vi "VisionExecute.v.vi"   [LabVIEW 2020]
uses:
  <vilib>/Rock Robotics/WPI/ThirdParty/PhotonPoseStrategy_ENUM.ctl
  <vilib>/Rock Robotics/WPI/ThirdParty/JAS_Junk/TrajLib/VI/Util_GetTime_U32.vi
  <vilib>/Rock Robotics/WPI/ThirdParty/PhotonVisionLib/SubVI/PhotonPipelineResult_CreateFromPacket.vi
  <vilib>/Rock Robotics/WPI/ThirdParty/PhotonVisionLib/SubVI/PhotonPipelineResult_SetTimeStampSecs.vi
  <vilib>/Rock Robotics/WPI/ThirdParty/PhotonVisionLib/SubVI/PhotonPipelineResult_GetLatency_Millis.vi
  <vilib>/Rock Robotics/WPI/ThirdParty/PhotonVisionLib/SubVI/PhotonPipelineResult_GetTimeStampSecs.vi
  <vilib>/Rock Robotics/WPI/ThirdParty/JAS_Junk/TrajLib/VI/Transform3d_Equals.vi
  <vilib>/Rock Robotics/WPI/ThirdParty/PhotonVisionLib/SubVI/PhotonPoseEstimator_SetStategy.vi
  <vilib>/Rock Robotics/WPI/ThirdParty/PhotonVisionLib/SubVI/PhotonPoseEstimator_SetHighestAmbiguity.vi
  <vilib>/Rock Robotics/WPI/ThirdParty/PhotonVisionLib/SubVI/PhotonPoseEstimator_New.vi
  <vilib>/Rock Robotics/WPI/ThirdParty/JAS_Junk/TrajLib/VI/AprilTagFieldLayout_NewSelect.vi
  <vilib>/Rock Robotics/WPI/ThirdParty/PhotonVisionLib/SubVI/PhotonPoseEstimator_SetLastPose.vi
  <vilib>/Rock Robotics/WPI/ThirdParty/PhotonVisionLib/SubVI/PhotonPoseEstimator_Update_PipeResult.vi
  <vilib>/Rock Robotics/WPI/ThirdParty/PhotonVisionLib/SubVI/PhotonPoseEstimator_SetReferencePose.vi
  <vilib>/Rock Robotics/WPI/ThirdParty/JAS_Junk/TrajLib/VI/Quaternion_New.vi
  <vilib>/Rock Robotics/WPI/ThirdParty/JAS_Junk/TrajLib/Conv_Deg_Radians.vi
  <vilib>/Rock Robotics/WPI/ThirdParty/JAS_Junk/TrajLib/VI/Pose3d_getTranslation3d.vi
  <vilib>/Rock Robotics/WPI/ThirdParty/JAS_Junk/TrajLib/VI/Pose3d_getRotation3d.vi
  <vilib>/Rock Robotics/WPI/ThirdParty/JAS_Junk/TrajLib/VI/Translation3d_ToTranslation2d.vi
  <vilib>/Rock Robotics/WPI/ThirdParty/JAS_Junk/TrajLib/VI/Rotation3d_ToRotation2d.vi
  <vilib>/Rock Robotics/WPI/ThirdParty/JAS_Junk/TrajLib/Pose2d_New_TRRO.vi
  <vilib>/Rock Robotics/WPI/ThirdParty/PhotonVisionLib/SubVI/Packet_decode_Flt64.vi
  <vilib>/Rock Robotics/WPI/ThirdParty/PhotonVisionLib/SubVI/Packet_decode_ByteI8.vi
  <vilib>/Rock Robotics/WPI/ThirdParty/PhotonVisionLib/SubVI/PhotonTrackedTarget_CreateFromPacket.vi
  <vilib>/Rock Robotics/WPI/ThirdParty/JAS_Junk/TrajLib/VI/Transform3d_GetTranslation3d.vi
  <vilib>/Rock Robotics/WPI/ThirdParty/JAS_Junk/TrajLib/VI/Transform3d_GetRotation3d.vi
  <vilib>/Rock Robotics/WPI/ThirdParty/JAS_Junk/TrajLib/VI/Rotation3d_Equals.vi
  <vilib>/Rock Robotics/WPI/ThirdParty/JAS_Junk/TrajLib/VI/Translation3d_Equals.vi
  <vilib>/Rock Robotics/WPI/ThirdParty/JAS_Junk/TrajLib/VI/AprilTagFieldLayout_New2022.vi
  <vilib>/Rock Robotics/WPI/ThirdParty/JAS_Junk/TrajLib/VI/AprilTagFieldLayout_New2023.vi
  <vilib>/Rock Robotics/WPI/ThirdParty/PhotonVisionLib/SubVI/PhotonPoseEstimator_GetEmptyPose.vi
  <vilib>/Rock Robotics/WPI/ThirdParty/PhotonVisionLib/SubVI/PhotonPoseEstimator_lowestAmbiguityStrategy.vi
  <vilib>/Rock Robotics/WPI/ThirdParty/PhotonVisionLib/SubVI/PhotonPoseEstimator_closestToCameraHeightStrategy.vi
  <vilib>/Rock Robotics/WPI/ThirdParty/PhotonVisionLib/SubVI/PhotonPoseEstimator_closestToReferencePoseStrategy.vi
  <vilib>/Rock Robotics/WPI/ThirdParty/PhotonVisionLib/SubVI/PhotonPoseEstimator_GetReferencePose.vi
  <vilib>/Rock Robotics/WPI/ThirdParty/PhotonVisionLib/SubVI/PhotonPoseEstimator_GetLastPose.vi
  <vilib>/Rock Robotics/WPI/ThirdParty/PhotonVisionLib/SubVI/PhotonPoseEstimator_averageBestTargetsStrategy.vi
  <vilib>/Rock Robotics/WPI/ThirdParty/JAS_Junk/TrajLib/Translation2d_Create.vi
  <vilib>/Rock Robotics/WPI/ThirdParty/JAS_Junk/TrajLib/Rotation2d_CreateAngle.vi
  <vilib>/Rock Robotics/WPI/ThirdParty/JAS_Junk/TrajLib/VI/Rotation3d_GetXYZ.vi
  <vilib>/Rock Robotics/WPI/ThirdParty/PhotonVisionLib/SubVI/TargetCorner_New.vi
  <vilib>/Rock Robotics/WPI/ThirdParty/PhotonVisionLib/SubVI/Packet_decode_Int32.vi
  <vilib>/Rock Robotics/WPI/ThirdParty/PhotonVisionLib/SubVI/Packet_decode_Transform3d.vi
  <vilib>/Rock Robotics/WPI/ThirdParty/JAS_Junk/TrajLib/VI/Rotation3d_GetQuaterion.vi
  <vilib>/Rock Robotics/WPI/ThirdParty/JAS_Junk/TrajLib/VI/Quaternion_Equals.vi
  <vilib>/Rock Robotics/WPI/ThirdParty/JAS_Junk/TrajLib/VI/AprilTagFieldLayout_New.vi
  <vilib>/Rock Robotics/WPI/ThirdParty/JAS_Junk/TrajLib/VI/Pose3d_New_Trans3dRot3d.vi
  <vilib>/Rock Robotics/WPI/ThirdParty/JAS_Junk/TrajLib/VI/Rotation3d_Create_Quaternion.vi
  <vilib>/Rock Robotics/WPI/ThirdParty/JAS_Junk/TrajLib/VI/AprilTag_New.vi
  <vilib>/Rock Robotics/WPI/ThirdParty/JAS_Junk/TrajLib/VI/Rotation3d_Create_AxisAngle.vi
  <vilib>/Rock Robotics/WPI/ThirdParty/JAS_Junk/TrajLib/VI/Pose3d_New.vi
  <vilib>/Rock Robotics/WPI/ThirdParty/PhotonVisionLib/SubVI/PhotonPipelineResult_HasTargets.vi
  <vilib>/Rock Robotics/WPI/ThirdParty/PhotonVisionLib/SubVI/PhotonEstimatedRobotPose_New.vi
  <vilib>/Rock Robotics/WPI/ThirdParty/PhotonVisionLib/SubVI/PhotonPipelineResult_GetTargets.vi
  <vilib>/Rock Robotics/WPI/ThirdParty/PhotonVisionLib/SubVI/PhotonTrackedTarget_GetPoseAmbiguity.vi
  <vilib>/Rock Robotics/WPI/ThirdParty/PhotonVisionLib/SubVI/PhotonTrackedTarget_GetFiducialId.vi
  <vilib>/Rock Robotics/WPI/ThirdParty/PhotonVisionLib/SubVI/PhotonPoseEstimator_GetFieldTags.vi
  <vilib>/Rock Robotics/WPI/ThirdParty/JAS_Junk/TrajLib/VI/AprilTagFieldLayout_GetTagPose.vi
  <vilib>/Rock Robotics/WPI/ThirdParty/JAS_Junk/TrajLib/VI/Pose3d_TransformBy.vi
  <vilib>/Rock Robotics/WPI/ThirdParty/PhotonVisionLib/SubVI/PhotonTrackedTarget_GetBestCameraToTarget.vi
  <vilib>/Rock Robotics/WPI/ThirdParty/JAS_Junk/TrajLib/VI/Transform3d_Inverse.vi
  <vilib>/Rock Robotics/WPI/ThirdParty/PhotonVisionLib/SubVI/PhotonPoseEstimator_GetHighestAmbiguity.vi
  <vilib>/Rock Robotics/WPI/ThirdParty/PhotonVisionLib/SubVI/PhotonPoseEstimator_GetRobotToCamera.vi
  <vilib>/Rock Robotics/WPI/ThirdParty/PhotonVisionLib/SubVI/PhotonPoseEstimator_closestToCameraHeightStrategy_calc.vi
  <vilib>/Rock Robotics/WPI/ThirdParty/PhotonVisionLib/SubVI/PhotonTrackedTarget_GetAltCameraToTarget.vi
  <vilib>/Rock Robotics/WPI/ThirdParty/PhotonVisionLib/SubVI/PhotonPoseEstimator_closestToReferencePoseStrategy_calc.vi
  <vilib>/Rock Robotics/WPI/ThirdParty/PhotonVisionLib/SubVI/PhotonPoseEstimator_averageBestTargetsStrategy_calc.vi
  <vilib>/Rock Robotics/WPI/ThirdParty/JAS_Junk/TrajLib/VI/Rotation3d_Plus.vi
  <vilib>/Rock Robotics/WPI/ThirdParty/JAS_Junk/TrajLib/VI/Translation3d_Plus.vi
  <vilib>/Rock Robotics/WPI/ThirdParty/JAS_Junk/TrajLib/VI/Translation3d_Times.vi
  <vilib>/Rock Robotics/WPI/ThirdParty/JAS_Junk/TrajLib/VI/Rotation3d_Times.vi
  <vilib>/Rock Robotics/WPI/ThirdParty/JAS_Junk/TrajLib/VI/Rotation3d_Create_Default.vi
  <vilib>/Rock Robotics/WPI/ThirdParty/JAS_Junk/TrajLib/VI/Translation3d_Create_Default.vi
  <vilib>/Rock Robotics/WPI/ThirdParty/JAS_Junk/TrajLib/VI/Quaternion_Get_All.vi
  <vilib>/Rock Robotics/WPI/ThirdParty/JAS_Junk/TrajLib/VI/Quaternion_Get_Vect.vi
  <vilib>/Rock Robotics/WPI/ThirdParty/JAS_Junk/TrajLib/VI/Quaternion_Get_W.vi
  <vilib>/Rock Robotics/WPI/ThirdParty/JAS_Junk/TrajLib/VI/AprilTag_GetAll.vi
  <vilib>/Rock Robotics/WPI/ThirdParty/JAS_Junk/TrajLib/VI/Quaternion_Normalize.vi
  <vilib>/Rock Robotics/WPI/ThirdParty/JAS_Junk/TrajLib/VI/Vector_Norm.vi
  <vilib>/Rock Robotics/WPI/ThirdParty/JAS_Junk/TrajLib/VecBuilder_ArrayBy1Fill.vi
  <vilib>/Rock Robotics/WPI/ThirdParty/JAS_Junk/TrajLib/VI/Pose3d_RelativeTo.vi
  <vilib>/Rock Robotics/WPI/ThirdParty/JAS_Junk/TrajLib/VI/Translation3d_RotateBy.vi
  <vilib>/Rock Robotics/WPI/ThirdParty/JAS_Junk/TrajLib/Transform2d_Create_TransRot.vi
  <vilib>/Rock Robotics/WPI/ThirdParty/JAS_Junk/TrajLib/VI/Rotation3d_UnaryMinus.vi
  <vilib>/Rock Robotics/WPI/ThirdParty/JAS_Junk/TrajLib/VI/Translation3d_UnaryMinus.vi
  <vilib>/Rock Robotics/WPI/ThirdParty/JAS_Junk/TrajLib/VI/Transform3d_GetXYZ.vi
  <vilib>/Rock Robotics/WPI/ThirdParty/JAS_Junk/TrajLib/VI/Pose3d_getXYZ.vi
  <vilib>/Rock Robotics/WPI/ThirdParty/PhotonVisionLib/SubVI/PhotonPoseEstimator_CalcDifference.vi
  <vilib>/Rock Robotics/WPI/ThirdParty/JAS_Junk/TrajLib/VI/Rotation3d_RotateBy.vi
  <vilib>/Rock Robotics/WPI/ThirdParty/JAS_Junk/TrajLib/VI/Translation3d_GetXYZ.vi
  <vilib>/Rock Robotics/WPI/ThirdParty/JAS_Junk/TrajLib/VI/Quaternion_New_Default.vi
  <vilib>/Rock Robotics/WPI/ThirdParty/JAS_Junk/TrajLib/MatBuilder_Create.vi
  <vilib>/Rock Robotics/WPI/ThirdParty/JAS_Junk/TrajLib/VI/Transform3d_Create_Pose3dPose3d.vi
  <vilib>/Rock Robotics/WPI/ThirdParty/JAS_Junk/TrajLib/VI/Quaternion_Times.vi
  <vilib>/Rock Robotics/WPI/ThirdParty/JAS_Junk/TrajLib/VI/Quaternion_Inverse.vi
  <vilib>/Rock Robotics/WPI/ThirdParty/JAS_Junk/TrajLib/VI/Translation3d_GetDistance.vi
  <vilib>/Rock Robotics/WPI/ThirdParty/JAS_Junk/TrajLib/VI/Translation3d_Minus.vi
  <vilib>/Rock Robotics/WPI/ThirdParty/JAS_Junk/TrajLib/VI/Rotation3d_Minus.vi
  <vilib>/Rock Robotics/SystemInterfaces/Utilities/FPGA_UtilitiesRead LocalTime.vi
  <vilib>/Rock Robotics/WPI/ThirdParty/JAS_Junk/TrajLib/VI/Util_GetTime_U64.vi
  <vilib>/Rock Robotics/Network Tables/NT Read Value.vi
  <vilib>/Rock Robotics/Network Tables/NT Read Raw.vi
  VisionGlobal.vi
  <vilib>/Rock Robotics/WPI/ThirdParty/JAS_Junk/TrajLib/Trajectory_Library.lvlib
  <vilib>/Rock Robotics/WPI/ThirdParty/PhotonVisionLib/PhotonVisionLib.lvlib
  <vilib>/Rock Robotics/WPI/ThirdParty/JAS_Junk/TrajLib/TypeDef/TRANSLATION2D.ctl
  <vilib>/Rock Robotics/WPI/ThirdParty/JAS_Junk/TrajLib/TypeDef/ROTATION2D.ctl
  <vilib>/Rock Robotics/WPI/ThirdParty/JAS_Junk/TrajLib/TypeDef/POSE2D.ctl
types:
  T1 = typedef "PhotonVisionLib.lvlib/PhotonPoseStrategy_ENUM.ctl" = enum16{"LOWEST_AMBIGUITY", "CLOSEST_TO_CAMERA_HEIGHT", "CLOSEST_TO_REFERENCE_POSE", "CLOSEST_TO_LAST_POSE", "AVERAGE_BEST_TARGETS"}
  T2 = typedef "Trajectory_Library.lvlib/TRANSLATION3D.ctl" = cluster{"X":dbl, "Y":dbl, "Z":dbl}
  T3 = typedef "Trajectory_Library.lvlib/ROTATION3D.ctl" = cluster{"Q_quaternion":T4}
  T4 = typedef "Trajectory_Library.lvlib/QUATERNION.ctl" = cluster{"R":dbl, "V":dbl[]}
  T5 = typedef "Trajectory_Library.lvlib/TRANSFORM3D.ctl" = cluster{"TRANSLATION3D":T2, "ROTATION3D":T3, "XF":bool}
  T6 = typedef "PhotonVisionLib.lvlib/PhotonPipelineResultType.ctl" = cluster{"TargetCount":i32, "Latency_MilliSec":dbl, "Targets":T7[], "TimeStampSec":dbl}
  T7 = typedef "PhotonVisionLib.lvlib/PhotonTrackedTargetType.ctl" = cluster{"Yaw":dbl, "Pitch":dbl, "Area":dbl, "Skew":dbl, "MinAreaRectCorners":T8[], "BestCameraToTarget":T5, "FiiducialId":i32, "AltCameraToTarget":T5, "PoseAmbiguity":dbl, "DetectedCorners":T8[]}
  T8 = typedef "PhotonVisionLib.lvlib/TargetCornerType.ctl" = cluster{"X":dbl, "Y":dbl}
  T9 = typedef "PhotonVisionLib.lvlib/PhotonPoseEstimator_Configuration.ctl" = cluster{"Strategy":T1, "Camera":string, "Initial Pose":T10, "AprilTagField":enum16{"2022 Rapid React", "2023 Charged Up"}, "HighestAmbiguity":dbl, "Use Custom Field":bool, "Custom AprilTag Field":T11, "RobotToCamera":T5}
  T10 = typedef "Trajectory_Library.lvlib/POSE3D.ctl" = cluster{"Translation3d":T2, "Rotation3d":T3}
  T11 = typedef "Trajectory_Library.lvlib/AprilTagFieldLayout.ctl" = cluster{"AprilTagMap":map{i32, T12}, "FieldLength":dbl, "FieldWidth":dbl, "OriginPosition ":T13, "OriginPose3d":T10}
  T12 = typedef "Trajectory_Library.lvlib/AprilTag.ctl" = cluster{"ID":i32, "POSE3D":T10}
  T13 = typedef "Trajectory_Library.lvlib/AprilTagFieldLayoutOrignPosition_ENUM.ctl" = enum16{"kBlueAllianceWallRightSide,", "kRedAllianceWallRightSide,"}
  T14 = typedef "PhotonVisionLib.lvlib/PhotonEstimatedRobotPoseType.ctl" = cluster{"EstimatedPose":T10, "TimeStamp_Seconds":dbl}
  T15 = typedef "Trajectory_Library.lvlib/POSE2D.ctl" = cluster{"TRANSLATION":T16, "ROTATION":T17}
  T16 = typedef "Trajectory_Library.lvlib/TRANSLATION2D.ctl" = cluster{"X":dbl, "Y":dbl}
  T17 = typedef "Trajectory_Library.lvlib/ROTATION2D.ctl" = cluster{"VALUE":dbl, "COS":dbl, "SIN":dbl}
  T18 = typedef "Trajectory_Library.lvlib/DIFF_DRIVE_POSE_EST2_CONFIG.ctl" = cluster{"TrackWidth_Meters":dbl, "Odom X std dev M":dbl, "Odom Y std dev M":dbl, "Odom Heading std dev Rad":dbl, "Vision X std dev M":dbl, "Vision Y std dev M":dbl, "Vision Heading std dev Rad":dbl}
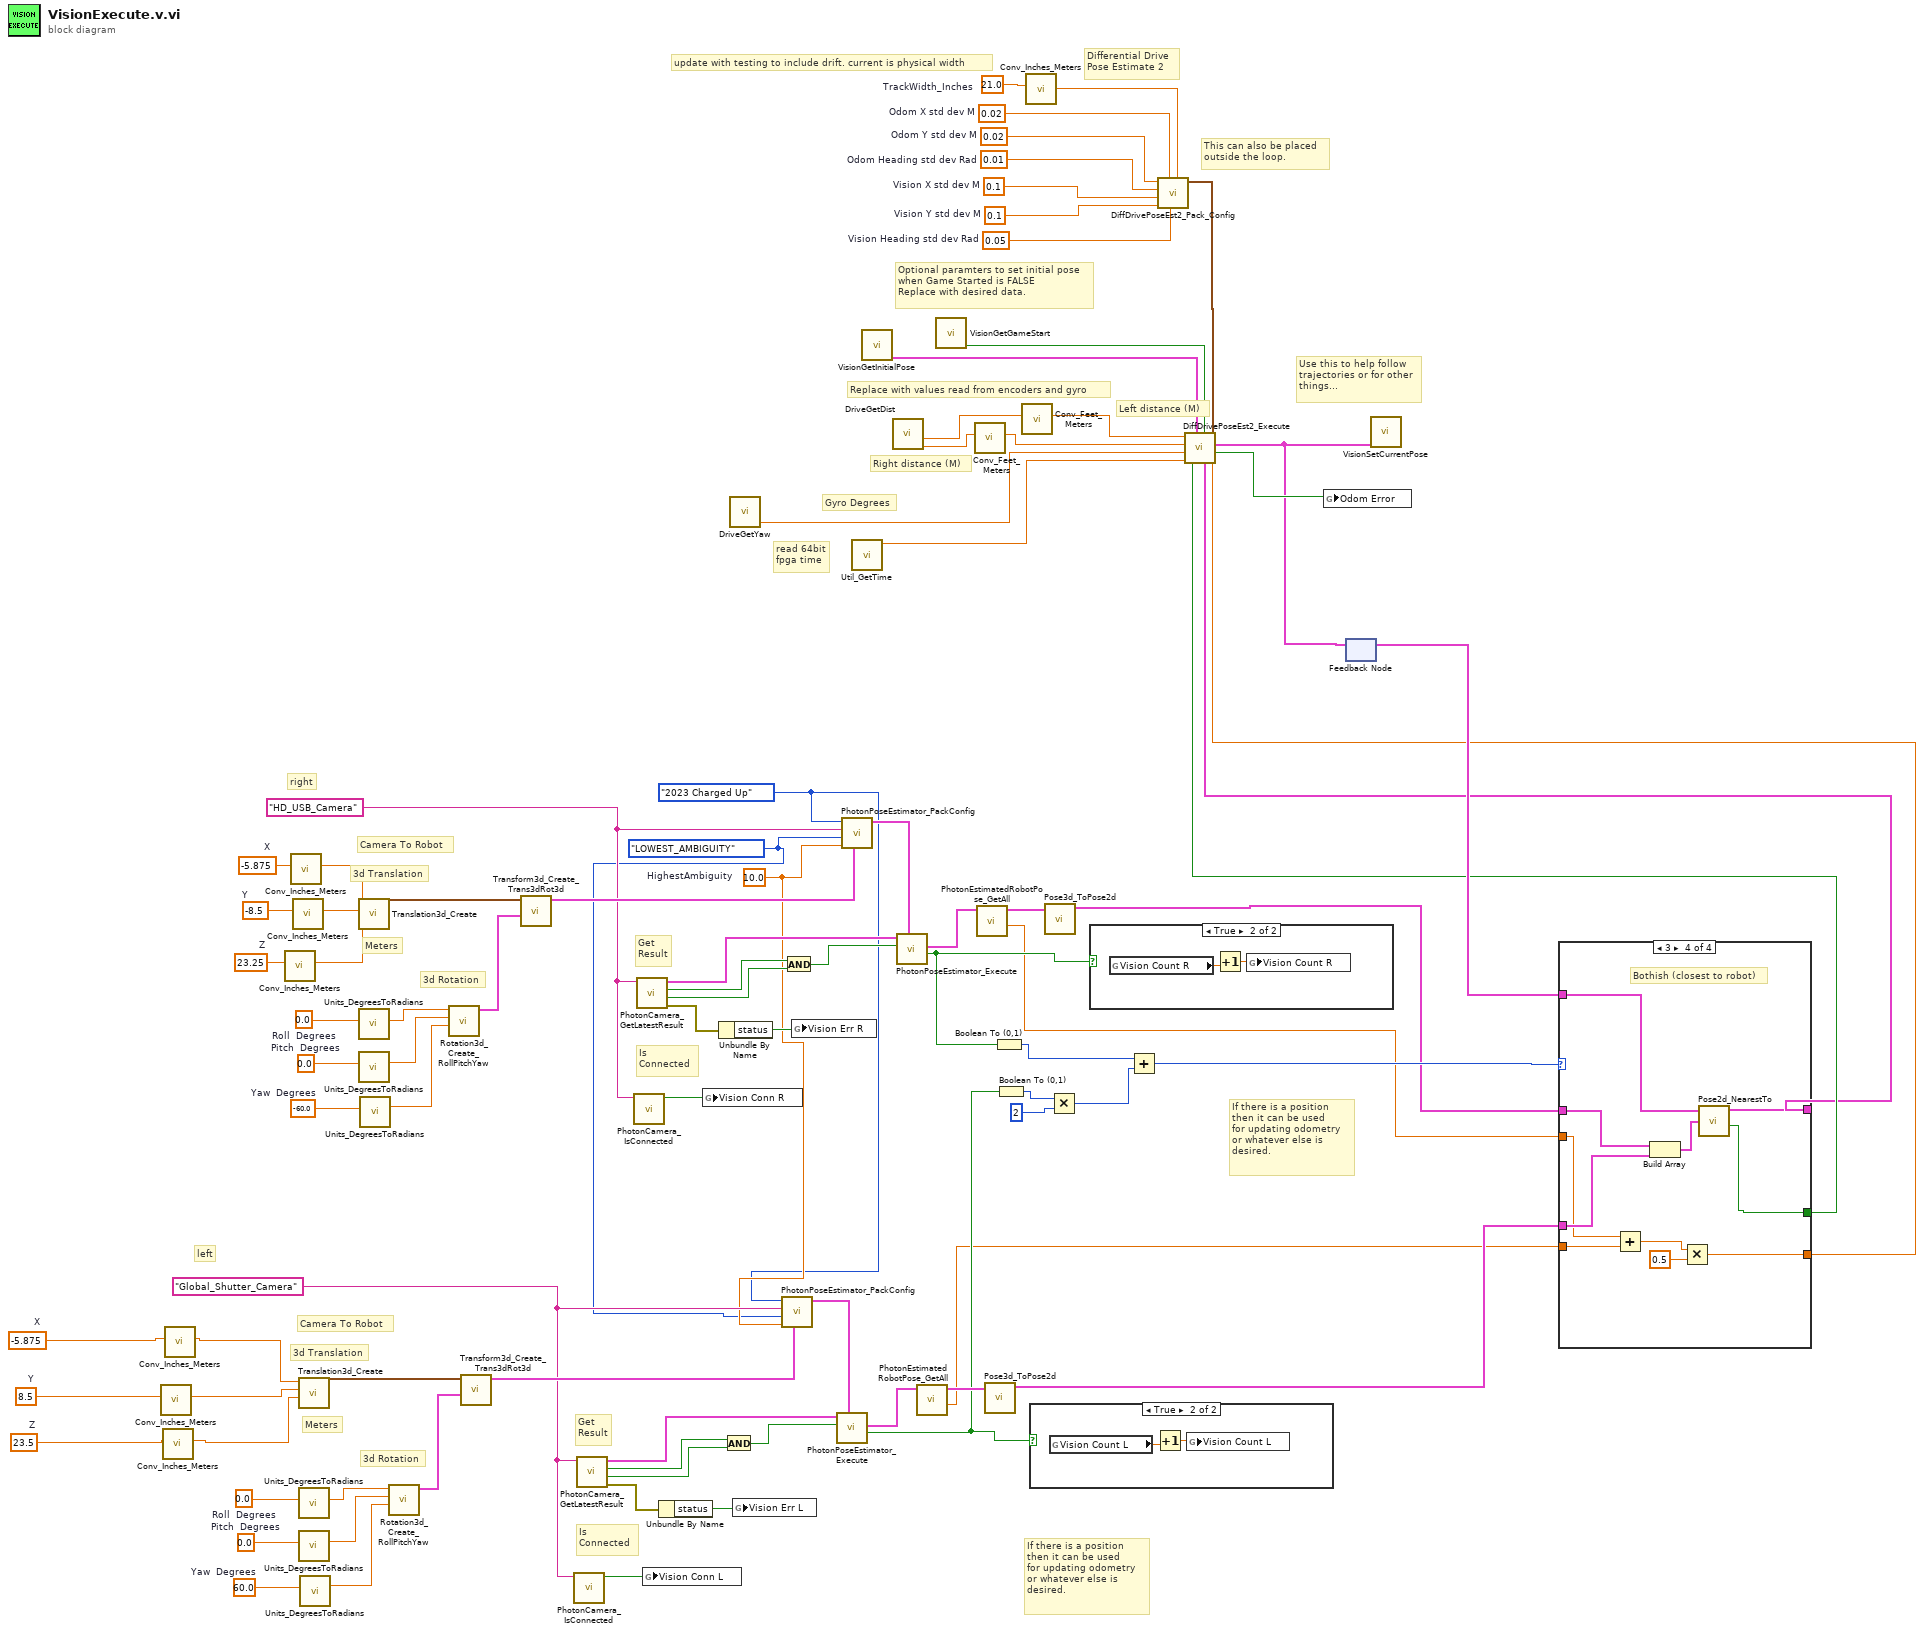
[diagram p0: block diagram]
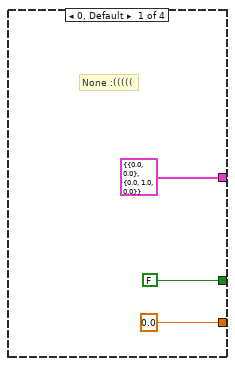
[diagram p2: hidden frame]
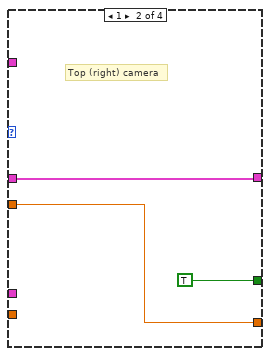
[diagram p3: hidden frame]
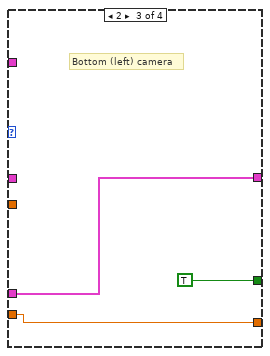
[diagram p4: hidden frame]
diagram:
  w44 = 0.0  # Roll  Degrees
  w43 = 0.0  # Pitch  Degrees
  w42 = 60.0  # Yaw  Degrees
  w27 = 23.5  # Z
  w31 = -5.875  # X
  w29 = 8.5  # Y
  w38 = "Global_Shutter_Camera" ("CameraName")
  w65 = 0.0  # Roll  Degrees
  w64 = 0.0  # Pitch  Degrees
  w63 = -60.0  # Yaw  Degrees
  w21 = 23.25  # Z
  w25 = -5.875  # X
  w23 = -8.5  # Y
  w19 = 10.0  # HighestAmbiguity
  w18 = PhotonPoseStrategy_ENUM."LOWEST_AMBIGUITY" ("Strategy")
  w17 = enum16{"2022 Rapid React", "2023 Charged Up"}."2023 Charged Up" ("AprilTagField")
  w59 = "HD_USB_Camera" ("CameraName")
  w81 = 21.0  # TrackWidth_Inches
  w83 = 0.02  # Odom Y std dev M
  w84 = 0.01  # Odom Heading std dev Rad
  w85 = 0.1  # Vision X std dev M
  w86 = 0.1  # Vision Y std dev M
  w87 = 0.02  # Odom X std dev M
  w88 = 0.05  # Vision Heading std dev Rad
  # "right"
  # "left"
  # "If there is a position\nthen it can be used\nfor updating odometry\nor whatever else is \ndesired."
  # "Meters"
  # "Camera To Robot"
  # "3d Rotation"
  # "3d Translation"
  # "Is\nConnected"
  # "Get\nResult"
  # "If there is a position\nthen it can be used\nfor updating odometry\nor whatever else is \ndesired."
  # "Meters"
  # "Camera To Robot"
  # "3d Rotation"
  # "3d Translation"
  # "Is\nConnected"
  # "Get\nResult"
  # "Gyro Degrees"
  # "Right distance (M)"
  # "Left distance (M)"
  # "update with testing to include drift. current is physical width"
  # "Replace with values read from encoders and gyro"
  # "Optional paramters to set initial pose\nwhen Game Started is FALSE\nReplace with desired data."
  # "read 64bit\nfpga time"
  # "This can also be placed \noutside the loop."
  # "Use this to help follow\ntrajectories or for other\nthings..."
  # "Differential Drive \nPose Estimate 2"
  n1 = call <vilib>:"Conv_Inches_Meters.vi"("INCH"=w29) -> ("Meters"=w28:dbl)  [unwired: 10 in]
  n2 = call <vilib>:"Conv_Inches_Meters.vi"("INCH"=w27) -> ("Meters"=w26:dbl)  [unwired: 10 in]
  n3 = call <vilib>:"Conv_Inches_Meters.vi"("INCH"=w31) -> ("Meters"=w30:dbl)  [unwired: 10 in]
  n4 = call <vilib>:"Conv_Inches_Meters.vi"("INCH"=w21) -> ("Meters"=w20:dbl)  [unwired: 10 in]
  n5 = call <vilib>:"Conv_Inches_Meters.vi"("INCH"=w25) -> ("Meters"=w24:dbl)  [unwired: 10 in]
  n6 = call <vilib>:"Conv_Inches_Meters.vi"("INCH"=w23) -> ("Meters"=w22:dbl)  [unwired: 10 in]
  n7 = call <vilib>:"Translation3d_Create.vi"("Z"=w26, "Y"=w28, "X"=w30) -> ("TRANSLATION3D"=w45:T2)  [unwired: 8 in]
  n8 = call <vilib>:"Units_DegreesToRadians.vi"("Degrees"=w44) -> ("Radians"=w41:dbl)  [unwired: 10 in]
  n9 = call <vilib>:"Units_DegreesToRadians.vi"("Degrees"=w43) -> ("Radians"=w40:dbl)  [unwired: 10 in]
  n10 = call <vilib>:"Units_DegreesToRadians.vi"("Degrees"=w42) -> ("Radians"=w39:dbl)  [unwired: 10 in]
  n11 = call <vilib>:"Translation3d_Create.vi"("Z"=w20, "Y"=w22, "X"=w24) -> ("TRANSLATION3D"=w66:T2)  [unwired: 8 in]
  n12 = call <vilib>:"Units_DegreesToRadians.vi"("Degrees"=w65) -> ("Radians"=w62:dbl)  [unwired: 10 in]
  n13 = call <vilib>:"Units_DegreesToRadians.vi"("Degrees"=w64) -> ("Radians"=w61:dbl)  [unwired: 10 in]
  n14 = call <vilib>:"Units_DegreesToRadians.vi"("Degrees"=w63) -> ("Radians"=w60:dbl)  [unwired: 10 in]
  n15 = call <vilib>:"Rotation3d_Create_RollPitchYaw.vi"("Yaw"=w39, "Pitch"=w40, "Roll"=w41) -> ("Rotation3d"=w46:T3)  [unwired: 8 in]
  n16 = call <vilib>:"Rotation3d_Create_RollPitchYaw.vi"("Yaw"=w60, "Pitch"=w61, "Roll"=w62) -> ("Rotation3d"=w67:T3)  [unwired: 8 in]
  n17 = call <vilib>:"Transform3d_Create_Trans3dRot3d.vi"("Rotation3d"=w46, "Translation3d"=w45) -> ("Transform3d"=w47:T5)  [unwired: 9 in]
  n18 = call <vilib>:"Transform3d_Create_Trans3dRot3d.vi"("Rotation3d"=w67, "Translation3d"=w66) -> ("Transform3d"=w68:T5)  [unwired: 9 in]
  n19 = call <vilib>:"PhotonCamera_IsConnected.vi"("CameraName"=w38) -> ("IsConnected"=w34:bool)  [unwired: 9 in, 1 out]
  n20 = call <vilib>:"PhotonCamera_GetLatestResult.vi"("CameraName"=w38) -> ("error out"=w33:errorcluster, "New Data"=w51:bool, "HasTargets"=w50:bool, "PipelineResult"=w48:T6)  [unwired: 7 in]
  n21 = call <vilib>:"PhotonCamera_IsConnected.vi"("CameraName"=w59) -> ("IsConnected"=w54:bool)  [unwired: 9 in, 1 out]
  n22 = call <vilib>:"PhotonCamera_GetLatestResult.vi"("CameraName"=w59) -> ("error out"=w53:errorcluster, "New Data"=w72:bool, "HasTargets"=w71:bool, "PipelineResult"=w69:T6)  [unwired: 7 in]
  n23 = global write "VisionGlobal.vi" "Vision Conn L"(w34) -> ()
  n24 = Unbundle By Name(w33) -> ("status"=w32:bool)
  n25 = global write "VisionGlobal.vi" "Vision Conn R"(w54) -> ()
  n26 = Unbundle By Name(w53) -> ("status"=w52:bool)
  n27 = And(x=w50, y=w51) -> (x .and. y?=w49:bool)
  n28 = call "DriveGetYaw.vi"() -> ("Yaw"=w75:dbl)  [unwired: 11 in]
  n29 = global write "VisionGlobal.vi" "Vision Err L"(w32) -> ()
  n30 = call <vilib>:"PhotonPoseEstimator_PackConfig.vi"("RobotToCamera"=w47, "HighestAmbiguity"=w19, "Strategy"=w18, "Camera"=w38, "AprilTagField"=w17) -> ("PoseEstimator_Configuration"=w37:T9)  [unwired: 6 in]
  n31 = And(x=w71, y=w72) -> (x .and. y?=w70:bool)
  n32 = global write "VisionGlobal.vi" "Vision Err R"(w52) -> ()
  n33 = call <vilib>:"PhotonPoseEstimator_Execute.vi"("Configuration"=w37, "PIpeline Has \nNew Results"=w49, "PipelineResult"=w48) -> ("Pos Found"=w14:bool, "PhotonEstimatedRobotPose"=w36:T14)  [unwired: 6 in, 1 out]
  n34 = call <vilib>:"PhotonPoseEstimator_PackConfig.vi"("RobotToCamera"=w68, "HighestAmbiguity"=w19, "Strategy"=w18, "Camera"=w59, "AprilTagField"=w17) -> ("PoseEstimator_Configuration"=w58:T9)  [unwired: 6 in]
  n35 = call <vilib>:"Util_GetTime.vi"() -> ("FPGA_Time_Seconds"=w82:dbl)  [unwired: 9 in, 2 out]
  n36 = call "VisionGetInitialPose.vi"() -> ("InitialPose"=w74:T15)  [unwired: 10 in]
  n37 = call "DriveGetDist.vi"() -> ("Right dist"=w79:dbl, "Left dist"=w78:dbl)  [unwired: 10 in]
  n38 = call <vilib>:"PhotonPoseEstimator_Execute.vi"("Configuration"=w58, "PIpeline Has \nNew Results"=w70, "PipelineResult"=w69) -> ("Pos Found"=w15:bool, "PhotonEstimatedRobotPose"=w57:T14)  [unwired: 6 in, 1 out]
  n39 = call <vilib>:"PhotonEstimatedRobotPose_GetAll.vi"("PhotonEstimatedRobotPose"=w36) -> ("TimeStamp_Seconds"=w4:dbl, "EstimatedPose"=w35:T10)  [unwired: 9 in]
  n40 = call "VisionGetGameStart.vi"() -> ("Game Start"=w73:bool)  [unwired: 11 in]
  n41 = call <vilib>:"Conv_Feet_Meters.vi"("Feet"=w79) -> ("Meters"=w76:dbl)  [unwired: 10 in]
  n42 = call <vilib>:"PhotonEstimatedRobotPose_GetAll.vi"("PhotonEstimatedRobotPose"=w57) -> ("TimeStamp_Seconds"=w5:dbl, "EstimatedPose"=w56:T10)  [unwired: 9 in]
  n43 = call <vilib>:"Pose3d_ToPose2d.vi"("in Pose3d"=w35) -> ("out Pose2d"=w7:T15)  [unwired: 10 in]
  n44 = Boolean To (0,1)(Boolean=w15) -> (0, 1=w10:i16)
  n45 = Boolean To (0,1)(Boolean=w14) -> (0, 1=w13:i16)
  n46 = call <vilib>:"Conv_Feet_Meters.vi"("Feet"=w78) -> ("Meters"=w77:dbl)  [unwired: 10 in]
  n47 = call <vilib>:"Conv_Inches_Meters.vi"("INCH"=w81) -> ("Meters"=w80:dbl)  [unwired: 10 in]
  n48 = case shown="True" w14 {
    frame False {
    }
    frame True {
      n49 = global read "VisionGlobal.vi" "Vision Count L"() -> (w90:dbl)
      n50 = Increment(x=w90) -> (x+1=w91:dbl)
      n51 = global write "VisionGlobal.vi" "Vision Count L"(w91) -> ()
    }
  }
  n52 = call <vilib>:"Pose3d_ToPose2d.vi"("in Pose3d"=w56) -> ("out Pose2d"=w8:T15)  [unwired: 10 in]
  n53 = Multiply(x=w13, y=i16 2) -> (x*y=w11:i16)
  n54 = case shown="True" w15 {
    frame False {
    }
    frame True {
      n55 = global read "VisionGlobal.vi" "Vision Count R"() -> (w92:dbl)
      n56 = Increment(x=w92) -> (x+1=w93:dbl)
      n57 = global write "VisionGlobal.vi" "Vision Count R"(w93) -> ()
    }
  }
  n58 = Add(x=w10, y=w11) -> (x+y=w9:i16)
  n59 = call <vilib>:"DiffDrivePoseEst2_Pack_Config.vi"("TrackWidth_Meters"=w80, "Vision Heading std dev Rad"=w88, "Odom X std dev M"=w87, "Vision Y std dev M"=w86, "Vision X std dev M"=w85, "Odom Heading std dev Rad"=w84, "Odom Y std dev M"=w83) -> ("DiffPoseEst2Config"=w89:T18)  [unwired: 4 in]
  n60 = feedback #1() -> (w6:T15)  [unwired: 1 in]
  n61 = case shown="3" w9 {
    tunnel: w8 -> [_ w98 _ w111]
    tunnel: w7 -> [_ _ w101 w110]
    tunnel: w6 -> [_ _ _ w112]
    tunnel: [FALSE ("Found") TRUE ("Found") TRUE ("Found") w108] -> w3
    tunnel: w5 -> [_ w99 _ w107]
    tunnel: w4 -> [_ _ w102 w106]
    tunnel: [T15 {"TRANSLATION"={"X"=0.0, "Y"=0.0}, "ROTATION"={"VALUE"=0.0, "COS"=1.0, "SIN"=0.0}} ("Nearest Pose") w98 w101 w109] -> w2
    tunnel: [0.0 w99 w102 w103] -> w1
    frame 0, Default {
      # "None :((((("
    }
    frame 1 {
      # "Top (right) camera"
    }
    frame 2 {
      # "Bottom (left) camera"
    }
    frame 3 {
      # "Bothish (closest to robot)"
      n62 = Add(x=w107, y=w106) -> (x+y=w105:dbl)
      n63 = Build Array(w111, w110) -> (w113:T15[])
      n64 = Multiply(x=w105, y=0.5) -> (x*y=w103:dbl)
      n65 = call <vilib>:"Pose2d_NearestTo.vi"("other POSE"=w113, "in POSE"=w112) -> ("Found"=w108:bool, "Nearest Pose"=w109:T15)  [unwired: 8 in]
    }
  }
  n66 = call <vilib>:"DiffDrivePoseEst2_Execute.vi"("Vision TImeStamp_Seconds"=w1, "DiffPoseEst2Config"=w89, "visionRobotPose"=w2, "Game Started"=w73, "Add Vision Meas"=w3, "InitialPose"=w74, "Pass Through Time"=w82, "Gyro Degrees"=w75, "RightDistance_M"=w76, "LeftDistance_M"=w77) -> ("Error"=w55:bool, "Estimated Pose"=w16:T15)
  n67 = global write "VisionGlobal.vi" "Odom Error"(w55) -> ()
  n68 = feedback-in #1(w16) -> ()
  n69 = call "VisionSetCurrentPose.vi"("Current Pose"=w16) -> ()  [unwired: 11 in]
